vi "Close Connection with CD.vi"(8 "error in":errorcluster, 11 "Connection Info":T1) -> (0 "error out":errorcluster)   [LabVIEW 2013, in "PID Control Host API.lvlib"]
uses:
  PID Control Host API.lvlib
  <userlib>/STM/TCP/stm_TCP Connection Info.ctl
  <userlib>/STM/_SubVIs/stm_MetaDataElement.ctl
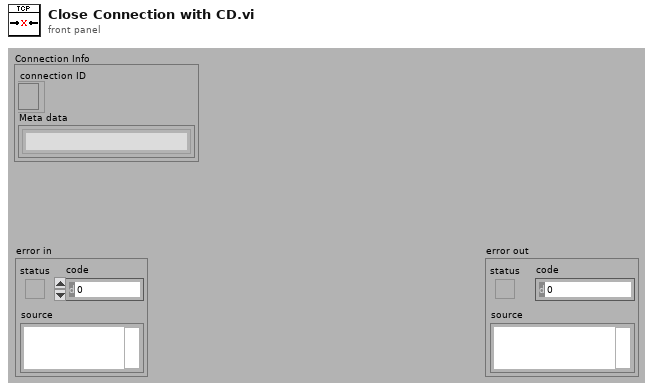
[diagram p1: front panel]
types:
  T1 = typedef "stm_TCP Connection Info.ctl" = cluster{"connection ID":refnum<k5>, "Meta data":T2[]}
  T2 = typedef "stm_MetaDataElement.ctl" = string
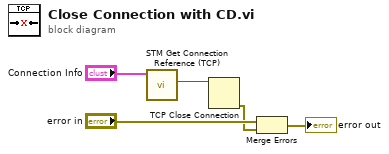
[diagram p0: block diagram]
diagram:
  n1 = call <userlib>:"STM Get Connection Reference (TCP).vi"("Connection Info"="Connection Info") -> ("connection ID out"=w4:refnum<k5>)  [unwired: 8 in, 2 out]
  n2 = TCP Close Connection(connection ID=w4) -> (error out=w2:errorcluster)  [unwired: 2 in, 1 out]
  n3 = Merge Errors("error in", w2) -> (→"error out":errorcluster)
